vi "Get Text File.vi"(8 "error in (no error)":errorcluster) -> (0 "error out":errorcluster, 2 "File Out":string)   [LabVIEW 2020, in "ATM Machine.lvlib"]
uses:
  ATM Machine.lvlib
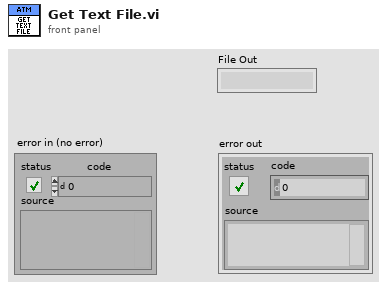
[diagram p1: front panel]
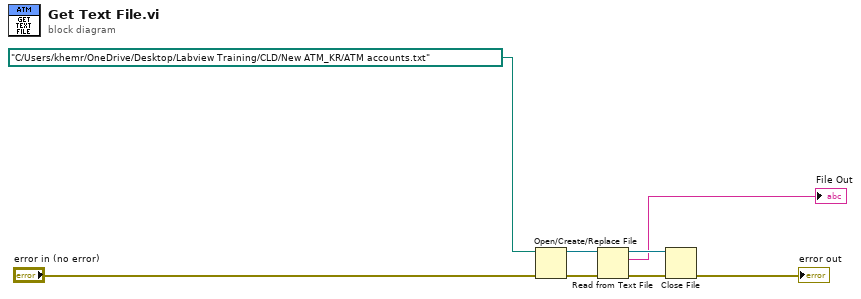
[diagram p0: block diagram]
diagram:
  n1 = Open/Create/Replace File(file path (use dialog)=path "C:/Users/khemr/OneDrive/Desktop/Labview Training/CLD/New ATM_KR/ATM accounts.txt", error in="error in (no error)") -> (refnum out=w5:refnum<file>, error out=w6:errorcluster)  [unwired: 4 in, 1 out]
  n2 = Read from Text File(file (use dialog)=w5, error in=w6) -> (refnum out=w2:refnum<file>, text=→"File Out":string, error out=w4:errorcluster)  [unwired: 2 in, 1 out]
  n3 = Close File(refnum=w2, error in=w4) -> (error out=→"error out":errorcluster)  [unwired: 1 out]
